vi "Config TDMS File for Asynchronous Write.vi"(8 "error in (no error)":errorcluster, 11 "base path":path=path "D:/USRP Project TDMS Files") -> (0 "error out":errorcluster, 3 "Refnum out":refnum<k34>)   [LabVIEW 2016]
doc: "Configure TDMS Settings for asynchronous write"
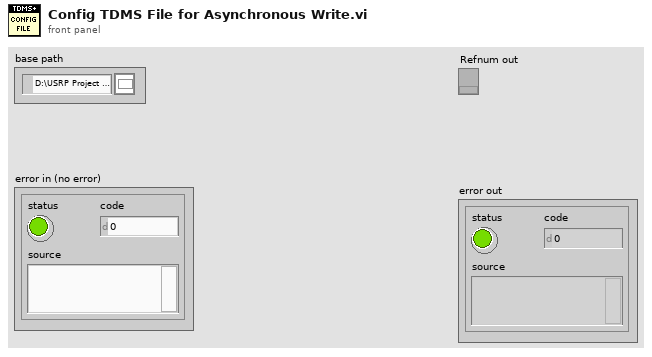
[diagram p1: front panel]
types:
  T1 = enum16{"open", "open or create", "create or replace", "create", "open (read-only)"}
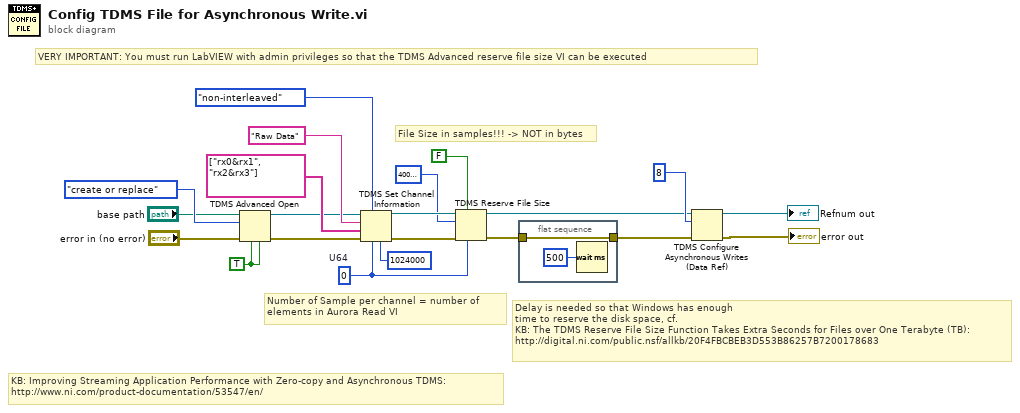
[diagram p0: block diagram]
diagram:
  w18 = u64 0  # U64
  w14 = TRUE ("enable asynchronous? (T)")
  # "KB: Improving Streaming Application Performance with Zero-copy and Asynchronous TDMS:\nhttp://www.ni.com/product-documentation/53547/en/"
  # "File Size in samples!!! -> NOT in bytes"
  # "Delay is needed so that Windows has enough \ntime to reserve the disk space, cf.\nKB: The TDMS Reserve File Size Function Takes Extra Seconds for Files over One Terabyte (TB): \nhttp://digital.ni.com/public.nsf/allkb/20F4FBCBEB3D553B86257B7200178683"
  # "VERY IMPORTANT: You must run LabVIEW with admin privileges so that the TDMS Advanced reserve file size VI can be executed"
  # "Number of Sample per channel = number of \nelements in Aurora Read VI"
  n1 = TDMS Advanced Open(4:w14, 6:w14, 8:"error in (no error)", 10:T1."create or replace" ("operation (0:open)"), 11:"base path") -> (0:w8:errorcluster, 3:w9:refnum<k34>)  [unwired: 1 out]
  n2 = TDMS Set Channel Information(4:u32 1024000 ("samples per channel"), 6:w18, 7:enum16{"non-interleaved", "interleaved"}."non-interleaved" ("data layout (0:non-interleaved)"), 8:w8, 9:string[] ["rx0&rx1", "rx2&rx3"] ("channel name(s)"), 10:"Raw Data" ("group name (Untitled)"), 11:w9) -> (0:w12:errorcluster, 3:w13:refnum<k34>)
  n3 = TDMS Reserve File Size(6:w18, 7:FALSE ("append? (T)"), 8:w12, 10:u64 40000000000 ("reserve size"), 11:w13) -> (0:w4:errorcluster, 3:w20:refnum<k34>)
  n4 = flat-sequence {
    tunnel: w4 -> [w23]
    tunnel: [w23] -> w3
    frame #0 {
      n5 = Wait (ms)(milliseconds to wait=u32 500) -> ()  [unwired: 1 out]
    }
  }
  n6 = TDMS Configure Asynchronous Writes (Data Ref)(8:w3, 10:u32 8 ("number of buffers (4)"), 11:w20) -> (0:→"error out":errorcluster, 3:→"Refnum out":refnum<k34>)  [unwired: 1 in]
